vi "Configure Output.vi"(6 "Operation Mode (0: Constant Current)":i32(ring) items=["Constant Current", "Constant Voltage"], 8 "error in (no error)":errorcluster, 9 "Output Voltage (0 V)":dbl, 10 "Output Current (0 A)":dbl, 11 "VISA resource name":refnum<visa-resource-name>) -> (0 "error out":errorcluster, 3 "VISA resource name out":refnum<visa-resource-name>)   [LabVIEW 2023]
doc: "Configures the output and operation mode of the instrument."
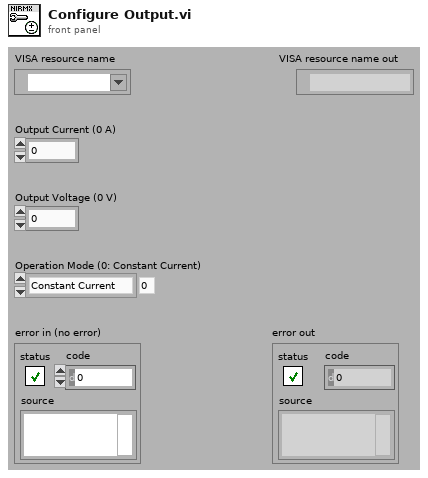
[diagram p1: front panel]
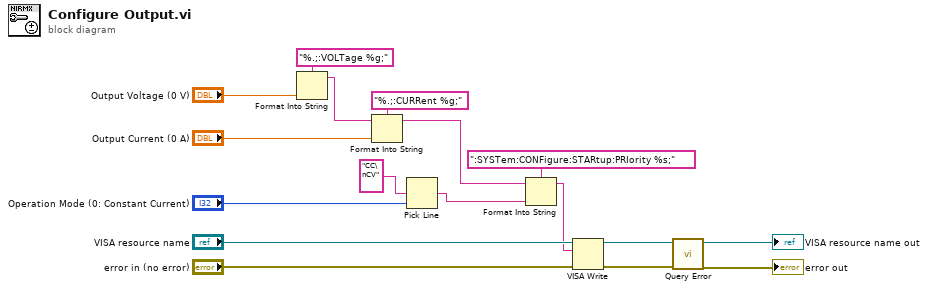
[diagram p0: block diagram]
diagram:
  n1 = Format Into String(format string="%.;:VOLTage %g;", "Output Voltage (0 V)") -> (resulting string=w15:string)  [unwired: 2 in, 1 out]
  n2 = Format Into String(format string="%.;:CURRent %g;", initial string=w15, "Output Current (0 A)") -> (resulting string=w2:string)  [unwired: 1 in, 1 out]
  n3 = Pick Line(multi-line string="CC\nCV", line index="Operation Mode (0: Constant Current)") -> (output string=w1:string)  [unwired: 1 in]
  n4 = Format Into String(format string=":SYSTem:CONFigure:STARtup:PRIority %s;", initial string=w2, w1) -> (resulting string=w3:string)  [unwired: 1 in, 1 out]
  n5 = VISA Write(VISA resource name="VISA resource name", write buffer=w3, error in (no error)="error in (no error)") -> (VISA resource name out=w10:refnum<visa-resource-name>, error out=w9:errorcluster)  [unwired: 1 out]
  n6 = call "Query Error.vi"("error in (no error)"=w9, "VISA resource name"=w10) -> ("error out"=→"error out":errorcluster, "VISA resource name out"=→"VISA resource name out":refnum<visa-resource-name>)  [unwired: 6 in, 2 out]
